vi "Call Subpanel VI.vi"(8 "error in (no error)":errorcluster, 10 "VI Refnum":refnum<vi>, 11 "Motions Configuration in":refnum<class "Motions Configuration.lvclass">) -> (0 "error out":errorcluster, 3 "Motions Configuration out":refnum<class "Motions Configuration.lvclass">)   [LabVIEW 2016, in "Hardware.lvlib" / "Motions.lvlib" / "Motions Configuration.lvclass"]
uses:
  <userlib>/Common Components/Hardware/Abstract System/Motions/Motions Config/Motions Configuration.lvclass
  <userlib>/Configuration Dialog Actor/Configuration.lvclass
  C:/Program Files (x86)/National Instruments/LabVIEW 2016/user.lib/Configuration Dialog Actor/Configuration.lvclass
  <userlib>/Configuration Dialog Actor/Configuration.lvclass/Configuration.ctl
  <vilib>/Utility/error.llb/Error Cluster From Error Code.vi
  <vilib>/ErrorRing/Error Ring.xnode
  <userlib>/Common Components/Hardware/Motor/Motor Config/Motor Configuration.lvclass
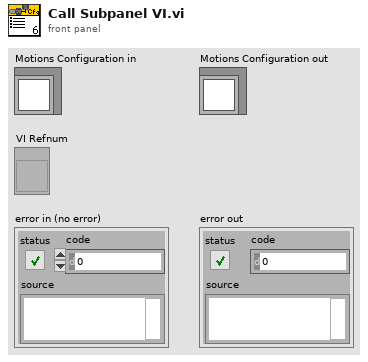
[diagram p1: front panel]
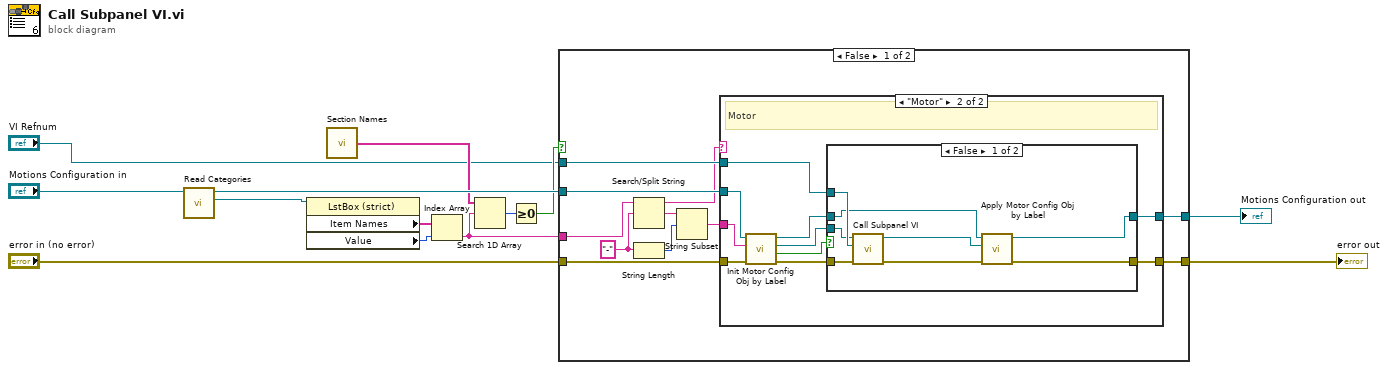
[diagram p0: block diagram]
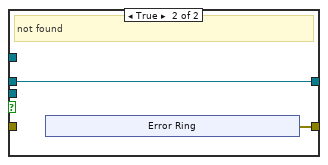
[diagram p3: hidden frame]
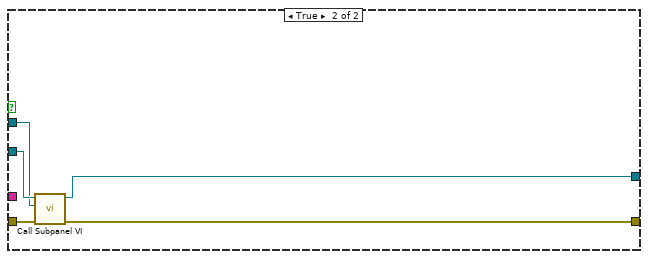
[diagram p4: hidden frame]
diagram:
  n1 = call <userlib>:"Read Categories.vi"("Configuration in"="Motions Configuration in") -> ("Categories"=w13:refnum<vi>, "Configuration out"=w10:refnum<class "Motions Configuration.lvclass">)  [unwired: 8 in, 1 out]
  n2 = property class="LstBox (strict)"(reference=w13) -> ("Item Names"=w11:string[], "Value"=w12:i32)  [unwired: 1 in, 2 out]
  n3 = call <userlib>:"Section Names.vi"() -> ("Array of Section Names"=w9:string[])
  n4 = Index Array(array=w11, index=w12) -> (element=w8:string)
  n5 = Search 1D Array(1D array=w9, element=w8) -> (index of element=w7:i32)  [unwired: 1 in]
  n6 = Greater Or Equal To 0?(x=w7) -> (x >= 0?=w6:bool)
  n7 = case shown="False" w6 {
    tunnel: "VI Refnum" -> [w24 w51]
    tunnel: "error in (no error)" -> [w23 w55]
    tunnel: [w22 w54] -> w2
    tunnel: [w21 w52] -> w3
    tunnel: w10 -> [w20 w53]
    tunnel: w8 -> [w19 _]
    frame False {
      w15 = "-" ("search string/char (-)")
      n8 = Search/Split String(string=w19, search string/char (-)=w15) -> (substring before match=w16:string, match + rest of string=w18:string)  [unwired: 1 in, 1 out]
      n9 = String Length(string=w15) -> (length=w17:i32)
      n10 = String Subset(string=w18, offset (0)=w17) -> (substring=w14:string)  [unwired: 1 in]
      n11 = case shown="\"Motor\"" w16 {
        tunnel: [w25 w31] -> w22
        tunnel: [w26 w29] -> w21
        tunnel: w23 -> [w25 w35]
        tunnel: w24 -> [_ w36]
        tunnel: w20 -> [w26 w34]
        tunnel: w14 -> [_ w28]
        frame Default {
        }
        frame "Motor" {
          # "Motor"
          n12 = call <userlib>:"Init Motor Config Obj by Label.vi"("error in (no error)"=w35, "Label"=w28, "Motions Configuration in"=w34) -> ("error out"=w33:errorcluster, "not found?"=w27:bool, "Motor Configuration Obj"=w32:refnum<class "Motor Configuration.lvclass">, "Motions Configuration out"=w30:refnum<class "Motions Configuration.lvclass">)  [unwired: 5 in]
          n13 = case shown="False" w27 {
            tunnel: w36 -> [w44 _]
            tunnel: w33 -> [w42 _]
            tunnel: w32 -> [w41 _]
            tunnel: [w40 w45] -> w31
            tunnel: w30 -> [w39 w46]
            tunnel: [w37 w46] -> w29
            frame False {
              n14 = call-dynamic "Call Subpanel VI.vi"("error in (no error)"=w42, "VI Refnum"=w44, "Motor Configuration in"=w41) -> ("error out"=w43:errorcluster, "Motor Configuration out"=w38:refnum<class "Motor Configuration.lvclass">)  [unwired: 7 in]
              n15 = call <userlib>:"Apply Motor Config Obj by Label.vi"("error in (no error)"=w43, "Motor Configuration Obj"=w38, "Motions Configuration in"=w39) -> ("error out"=w40:errorcluster, "Motions Configuration out"=w37:refnum<class "Motions Configuration.lvclass">)  [unwired: 7 in]
            }
            frame True {
              # "not found"
              n16 = xnode "Error Ring"() -> ("error out"=w45:errorcluster)
            }
          }
        }
      }
    }
    frame True {
      n17 = call-parent "Call Subpanel VI.vi"("error in (no error)"=w55, "VI Refnum"=w51, "Configuration in"=w53) -> ("error out"=w54:errorcluster, "Configuration out"=w52:refnum<class "Motions Configuration.lvclass">)  [unwired: 7 in]
    }
  }
  "error out" <- w2
  "Motions Configuration out" <- w3
